vi "Pose3d_Equals.vi"(9 "other Pose3d":T1={"Translation3d"={"X"=0.0, "Y"=0.0, "Z"=0.0}, "Rotation3d"={"Q_quaternion"={"R"=1.0, "V"=[0.0, 0.0, 0.0]}}} {"Translation3d"."Z" format="%14.3f"; "Translation3d"."Y" format="%14.3f"; "Translation3d"."X" format="%14.3f"}, 11 "in Pose3d":T1={"Translation3d"={"X"=0.0, "Y"=0.0, "Z"=0.0}, "Rotation3d"={"Q_quaternion"={"R"=1.0, "V"=[0.0, 0.0, 0.0]}}} {"Translation3d"."Z" format="%14.3f"; "Translation3d"."Y" format="%14.3f"; "Translation3d"."X" format="%14.3f"}) -> (3 "Equals":bool)   [LabVIEW 2019, in "Trajectory_Library.lvlib"]
doc: "Checks equality between this Pose3d and another Pose3d.\n\nParameters:\n - this Pose3d - This POSE3D data structure\n - other POSE3d - The other POSE23 data structure\n\nReturns: \n - Equals - Value will be TRUE if both POSEs are the same"
uses:
  Trajectory_Library.lvlib
  TypeDef/TRANSLATION3D.ctl
  TypeDef/QUATERNION.ctl
  TypeDef/ROTATION3D.ctl
  POSE3D.ctl
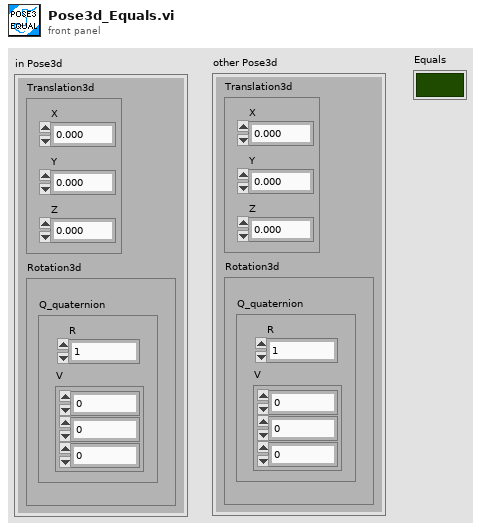
[diagram p1: front panel]
types:
  T1 = typedef "Trajectory_Library.lvlib/POSE3D.ctl" = cluster{"Translation3d":T2, "Rotation3d":T3}
  T2 = typedef "Trajectory_Library.lvlib/TRANSLATION3D.ctl" = cluster{"X":dbl, "Y":dbl, "Z":dbl}
  T3 = typedef "Trajectory_Library.lvlib/ROTATION3D.ctl" = cluster{"Q_quaternion":T4}
  T4 = typedef "Trajectory_Library.lvlib/QUATERNION.ctl" = cluster{"R":dbl, "V":dbl[]}
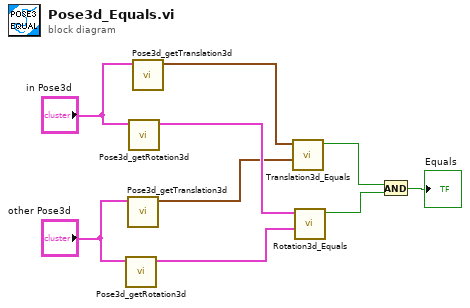
[diagram p0: block diagram]
diagram:
  n1 = call "Pose3d_getRotation3d.vi"("in Pose3d"="other Pose3d") -> ("out Rotation3d"=w1:T3)  [unwired: 10 in]
  n2 = call "Pose3d_getTranslation3d.vi"("in Pose3d"="other Pose3d") -> ("out Translation3d"=w3:T2)  [unwired: 10 in]
  n3 = call "Pose3d_getRotation3d.vi"("in Pose3d"="in Pose3d") -> ("out Rotation3d"=w5:T3)  [unwired: 10 in]
  n4 = call "Pose3d_getTranslation3d.vi"("in Pose3d"="in Pose3d") -> ("out Translation3d"=w2:T2)  [unwired: 10 in]
  n5 = call "Translation3d_Equals.vi"("other Translation3d"=w3, "In Translation3d"=w2) -> ("Equals"=w8:bool)  [unwired: 9 in]
  n6 = call "Rotation3d_Equals.vi"("other Rotation3d"=w1, "in Rotation3d"=w5) -> ("Equals"=w7:bool)  [unwired: 9 in]
  n7 = And(x=w8, y=w7) -> (x .and. y?=→"Equals":bool)
